vi "PART_II.vi"() -> ()   [LabVIEW 2019]
uses:
  <vilib>/Utility/file.llb/Read Delimited Spreadsheet (DBL).vi
panel:
  in  "n-points after peak":i32
  in  "n-points before peak":i32
  out "Trigger Plot":dbl[](graph)
  out "Original Signal":dbl(graph)
  out "all rows":dbl[][](array[numeric])
  in  "threshold":dbl
  out "subarray":dbl[](array[numeric])
  in  "file path (dialog if empty)":path
  in  "stop":bool
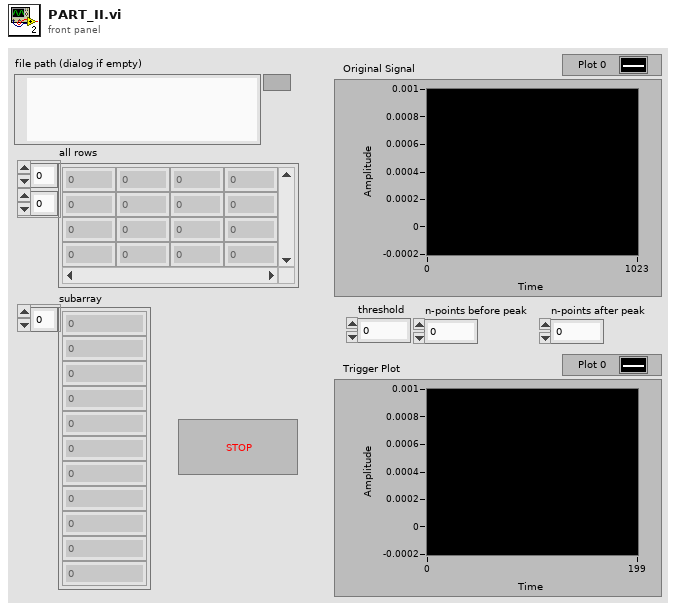
[diagram p1: front panel]
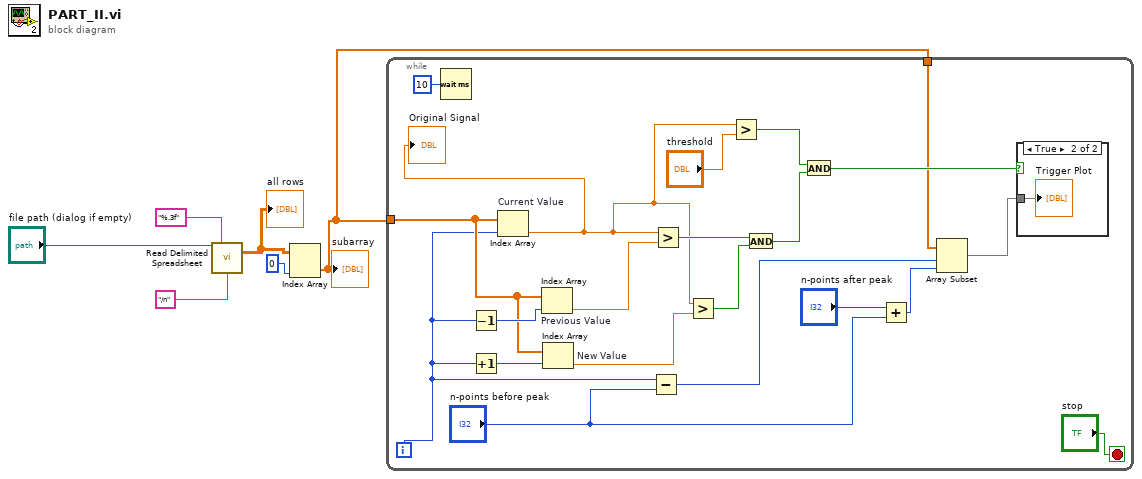
[diagram p0: block diagram]
diagram:
  n1 = call-poly <vilib>:"Read Delimited Spreadsheet.vi"("file path (dialog if empty)"="file path (dialog if empty)", "format (%.3f)"="%.3f", "delimiter (\\t)"="/n" ("delimiter (\\t)")) -> ("all rows"=w3:dbl[][])  [unwired: 7 in, 5 out]
  "all rows" <- w3
  n2 = Index Array(array=w3, index (col)=0 ("disabled index (col)")) -> (element=w1:dbl[])  [unwired: 1 in]
  "subarray" <- w1
  n3 = while {
    tunnel: w1 -> [w15]
    tunnel: w1 -> [w7]
    i -> [w13]
    stop <- "stop" stop-if-true
    n4 = Wait (ms)(milliseconds to wait=u32 10) -> ()  [unwired: 1 out]
    n5 = Decrement(x=w13) -> (x-1=w25:i32)
    n6 = Increment(x=w13) -> (x+1=w24:i32)
    n7 = Index Array "Current Value"(array=w15, index=w13) -> (element=w14:dbl)
    "Original Signal" <- w14
    n8 = Index Array "Previous Value"(array=w15, index=w25) -> (element=w23:dbl)
    n9 = Index Array "New Value"(array=w15, index=w24) -> (element=w22:dbl)
    n10 = Subtract(x=w13, y="n-points before peak") -> (x-y=w12:i32)
    n11 = Greater?(x=w14, y=w23) -> (0:w20:bool)
    n12 = Greater?(x=w14, y=w22) -> (0:w19:bool)
    n13 = Greater?(x=w14, y="threshold") -> (0:w18:bool)
    n14 = And(x=w20, y=w19) -> (x .and. y?=w17:bool)
    n15 = And(x=w18, y=w17) -> (x .and. y?=w16:bool)
    n16 = Add(x="n-points after peak", y="n-points before peak") -> (x+y=w10:i32)
    n17 = Array Subset "Array Subset"(array=w7, index=w12, length=w10) -> (w11:dbl[])
    n18 = case shown="True" w16 {
      tunnel: w11 -> [_ w28]
      frame False {
      }
      frame True {
        "Trigger Plot" <- w28
      }
    }
  }
